vi "modeControls.vi"(8 "error in (no error)":errorcluster, 10 "Enabled/Disabled":T1(ring), 11 "SR430Class in":refnum<class "SR430Class.lvclass">) -> (0 "error out":errorcluster, 3 "SR430Class out":refnum<class "SR430Class.lvclass">)   [LabVIEW 2015, in "SR430Class.lvclass"]
uses:
  class/SR430Class.lvclass
  class/SR430Class.lvclass/SR430Class.ctl
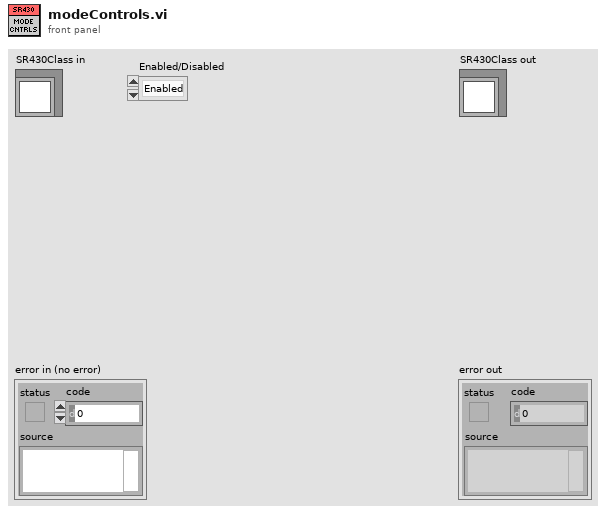
[diagram p1: front panel]
types:
  T1 = enum8{"Enabled", "Disabled", "Disabled and Grayed Out"}
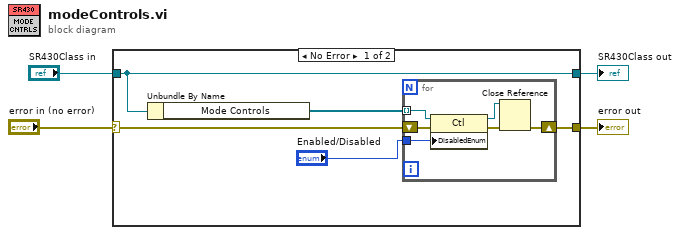
[diagram p0: block diagram]
diagram:
  n1 = case shown="No Error" "error in (no error)" {
    selector: "error in (no error)" -> [w9 w17]
    tunnel: [w8 w17] -> w3
    tunnel: [w7 w16] -> w1
    tunnel: "SR430Class in" -> [w7 w16]
    frame No Error {
      n2 = Unbundle By Name(w7) -> ("Mode Controls"=w6:refnum<vi>[])
      n3 = for {
        tunnel: "Enabled/Disabled" -> [w15]
        shift-right: [w11] -> w8
        shift-left: w9 -> [w14]
        tunnel: w6 -> [w10] mode=indexing
        n4 = property class="Ctl"(reference=w10, error in=w14, "DisabledEnum"=w15) -> (reference out=w13:refnum<vi>, error out=w12:errorcluster)
        n5 = Close Reference(reference=w13, error in (no error)=w12) -> (error out=w11:errorcluster)
      }
    }
    frame Error {
    }
  }
  "error out" <- w3
  "SR430Class out" <- w1
